vi "UDP2File.vi"() -> ()   [LabVIEW 2012]
panel:
  out "String":string
  out "packet in \nconstruction":u32
  out "packet constructed":u32
  out "UDP reciever\nloop":u32
  out "start time":u32
  out "channel":u32
  out "Found Header":bool
  out "Raw Data Out":string
  out "error post-check":errorcluster
  out "End Reciever Error":errorcluster
  in  "stop reciever":bool
  out "port":u16
  out "error out post-read":errorcluster
  out "error out pre-read":errorcluster
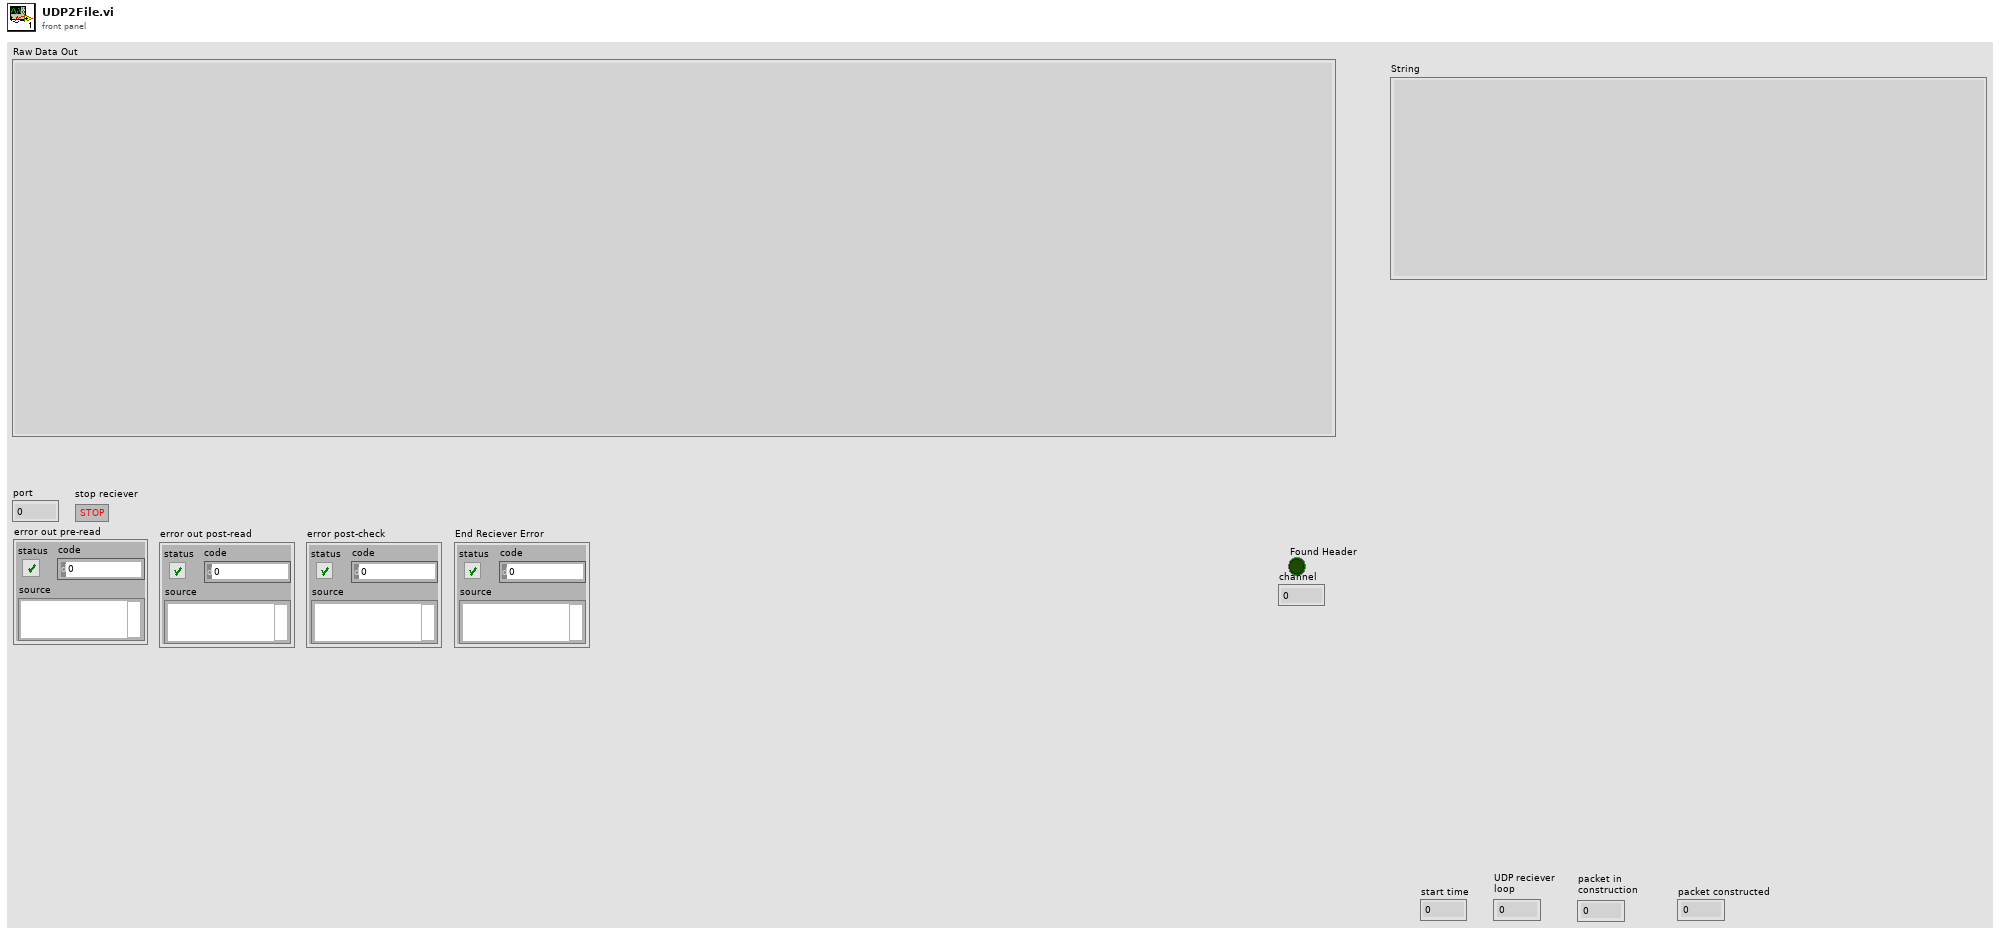
[diagram p1: front panel]
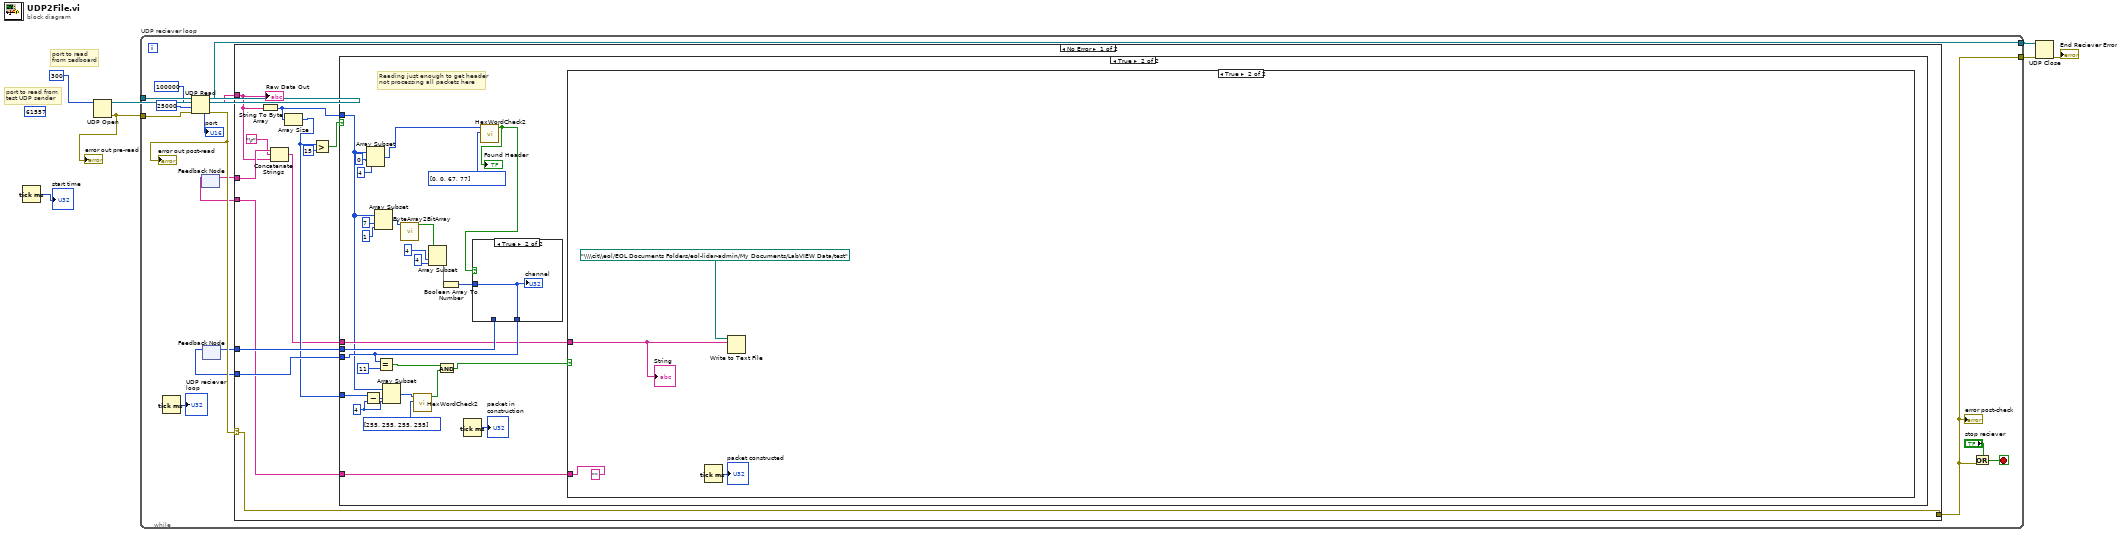
[diagram p0: block diagram]
diagram:
  (unwired) u16 61557 ("port")
  # "port to read \nfrom zedboard"
  # "port to read from \ntest UDP sender"
  n1 = Tick Count (ms)() -> (millisecond timer value=→"start time":u32)
  n2 = UDP Open(11:u16 300 ("port")) -> (port=w6:refnum<k16>, 0:w3:errorcluster)  [unwired: 4 in, 1 out]
  "error out pre-read" <- w3
  n3 = while "UDP reciever loop" {
    tunnel: [w23] -> w7
    tunnel: w6 -> [w22]
    tunnel: [w14] -> w5
    tunnel: w3 -> [w19]
    stop <- w21 stop-if-true
    n4 = Tick Count (ms)() -> (millisecond timer value=→"UDP reciever\nloop":u32)
    n5 = UDP Read(connection ID=w22, max size (548)=100000, timeout ms (25000)=25000, 8:w19) -> (data out=w16:string, error out=w18:errorcluster, 3:w23:refnum<k16>, 4:→"port":u16)  [unwired: 1 out]
    "error out post-read" <- w18
    n6 = feedback #1() -> (w11:string)  [unwired: 1 in]
    n7 = feedback #2() -> (w9:u32)  [unwired: 1 in]
    n8 = case shown="No Error" w18 {
      selector: w18 -> [w35 w75]
      tunnel: w16 -> [w24 _]
      tunnel: [w35 w75] -> w14
      tunnel: [w29 w74] -> w12
      tunnel: w11 -> [w26 w74]
      tunnel: [w32 w73] -> w10
      tunnel: w9 -> [w31 w73]
      frame No Error {
        n9 = String To Byte Array(string=w24) -> (unsigned byte array=w30:u8[])
        n10 = Concatenate Strings(w26, "\r", w24) -> (w27:string)
        n11 = Array Size(array=w30) -> (size(s)=w28:i32)
        n12 = Greater?(x=w28, y=15) -> (0:w34:bool)
        n13 = case shown="True" w34 {
          tunnel: w30 -> [_ w47]
          tunnel: [w37 w51] -> w32
          tunnel: w31 -> [w37 w52]
          tunnel: w28 -> [_ w55]
          tunnel: w27 -> [w36 w49]
          tunnel: [w36 w48] -> w29
          frame False {
          }
          frame True {
            w57 = 4 ("length")
            # "Reading just enough to get header\nnot processing all packets here"
            n14 = Subtract(x=w55, y=w57) -> (x-y=w56:i32)
            n15 = Array Subset(array=w47, index=0, length=4) -> (w61:u8[])
            n16 = Array Subset(array=w47, index=7, length=1) -> (w44:u8[])
            n17 = Array Subset(array=w47, index=w56, length=w57) -> (w50:u8[])
            n18 = call "ByteArray2BitArray.vi"("array"=w44) -> ("Array"=w41:bool[])  [unwired: 10 in]
            n19 = call "HexWordCheck2.vi"("array"=u8[] [255, 255, 255, 255], "Input Array"=w50) -> ("Boolean"=w58:bool)  [unwired: 9 in]
            n20 = Array Subset(array=w41, index=4, length=4) -> (w39:bool[])
            n21 = Boolean Array To Number(Boolean array=w39) -> (number=w40:u32)
            n22 = Tick Count (ms)() -> (millisecond timer value=→"packet in \nconstruction":u32)
            n23 = call "HexWordCheck2.vi"("array"=u8[] [0, 0, 67, 77], "Input Array"=w61) -> ("Boolean"=w62:bool)  [unwired: 9 in]
            "Found Header" <- w62
            n24 = case shown="True" w62 {
              tunnel: [w71 w72] -> w51
              tunnel: w52 -> [w71 _]
              tunnel: w40 -> [_ w72]
              frame False {
              }
              frame True {
                "channel" <- w72
              }
            }
            n25 = Equal?(x=w51, y=u32 11) -> (x = y?=w54:bool)
            n26 = And(x=w54, y=w58) -> (x .and. y?=w59:bool)
            n27 = case shown="True" w59 {
              tunnel: w49 -> [w66 w67]
              tunnel: [w66 ""] -> w48
              frame False {
              }
              frame True {
                n28 = Tick Count (ms)() -> (millisecond timer value=→"packet constructed":u32)
                n29 = Write to Text File(file (use dialog)=path "\\\\cit\\eol/EOL Documents Folders/eol-lidar-admin/My Documents/LabVIEW Data/test", text=w67) -> ()  [unwired: 2 in, 3 out]
                "String" <- w67
              }
            }
          }
        }
        "Raw Data Out" <- w24
      }
      frame Error {
      }
    }
    "error post-check" <- w14
    n30 = feedback-in #1(w12) -> ()
    n31 = feedback-in #2(w10) -> ()
    n32 = Or(x="stop reciever", y=w14) -> (x .or. y?=w21:bool)
  }
  n33 = UDP Close(connection ID=w7, 8:w5) -> (error out=→"End Reciever Error":errorcluster)  [unwired: 1 out]
